vi "Close.vi"(0 "connection ID":refnum<k5>, 5 "error in":errorcluster) -> (19 "error out":errorcluster)   [LabVIEW 2010, in "RedPitaya.lvlib"]
doc: "Terminates the software connection to Red Pitaya."
uses:
  RedPitaya.lvlib
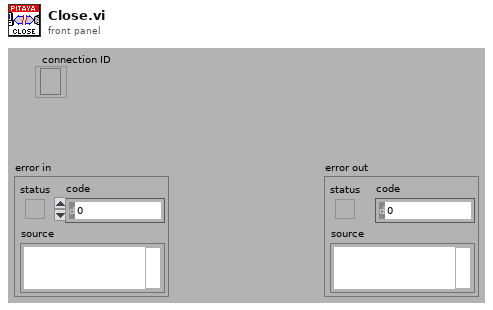
[diagram p1: front panel]
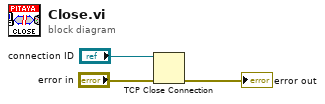
[diagram p0: block diagram]
diagram:
  n1 = TCP Close Connection(connection ID="connection ID", error in (no error)="error in") -> (error out=→"error out":errorcluster)  [unwired: 1 in, 1 out]
